vi "processSubDataPublish.vi"(8 "error in (no error)":errorcluster, 11 "MiddlewareSALThisComponent in":refnum<class "MiddlewareSALThisComponent.lvclass">) -> (0 "error out":errorcluster, 3 "MiddlewareSALThisComponent out":refnum<class "MiddlewareSALThisComponent.lvclass">)   [LabVIEW 2016, in "MiddlewareSALThisComponent.lvclass"]
uses:
  MiddlewareSALThisComponent.lvclass
  home/harini/tcs/ts_sedspectrometer/ComponentTemplateCore/ComponentModel/ComponentModel/Middleware/Middleware.lvclass
  ComponentTemplateCore/ComponentModel/ComponentModel/Middleware/Middleware.lvclass/Middleware.ctl
  ComponentTemplateCore/ComponentModel/ComponentModel/MiddlewareProcessEvent/MiddlewareProcessEvent.lvclass/MiddlewareProcessEvent.ctl
  MiddlewareSALThisComponent.lvclass/MiddlewareSALThisComponent.ctl
  PubSubDataEvent/PubSubDataEvent.lvclass/PubSubDataEvent.ctl
  <vilib>/Utility/error.llb/DialogType.ctl
  Typedefs/SubDataSignal.ctl
  ts_sallv_sedspectrometer/DataTypes/command_CaptureSpectImage.ctl
  ts_sallv_sedspectrometer/DataTypes/command_SetSpectTempSetpoint.ctl
  ts_sallv_sedspectrometer/DataTypes/command_StopImageCapture.ctl
  Typedefs/EXATypedefs.lvlib
  ComponentTemplateCore/ComponentModel/ComponentModel/Middleware/Middleware.lvclass
  ComponentTemplateCore/ComponentModel/ComponentModel/MiddlewareProcessEvent/MiddlewareProcessEvent.lvclass
  PubSubDataEvent/PubSubDataEvent.lvclass
  ProgrammaticInitialization/ProgrammaticInitialization.lvclass
  ts_sallv_sedspectrometer/SALLV_calibrationSpectrometer.lvlib
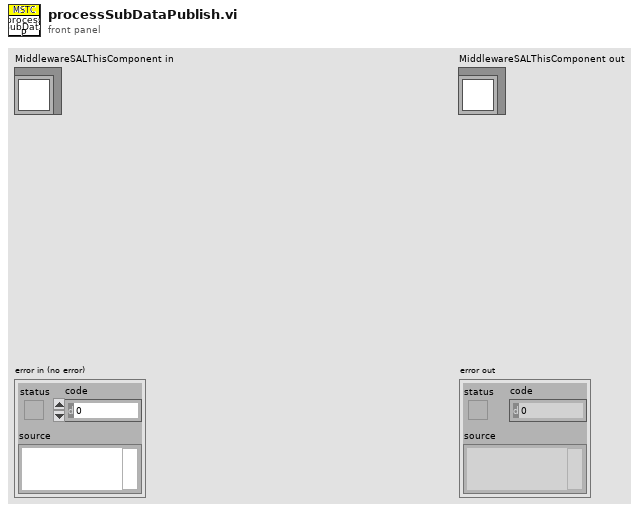
[diagram p1: front panel]
types:
  T1 = typedef "TypedefsDataEvents.lvlib/SubDataEvents.ctl" = cluster{"Disable":refnum<user-event>, "Enable":refnum<user-event>, "ExitControl":refnum<user-event>, "Standby":refnum<user-event>, "Heartbeat":refnum<user-event>, "Start":refnum<user-event>, "CaptureSpectImage":refnum<user-event>, "SetSpectTempSetpoint":refnum<user-event>, "StopImageCapture":refnum<user-event>}
  T2 = typedef "MiddlewareProcessEvents.ctl" = cluster{"disconnect":refnum<user-event>, "error":refnum<user-event>}
  T3 = typedef "EXATypedefs.lvlib/SubDataSignal.ctl" = enum16{"Disable", "Enable", "Exit", "GoToStandby", "HeartbeatIn", "Start", "CaptureSpectImage", "SetSpectTempSetpoint", "StopImageCapture"}
  T4 = typedef "SALLV_calibrationSpectrometer.lvlib/command_CaptureSpectImage.ctl" = cluster{"spectId":u16, "intTime":sgl, "intDelay":dbl, "numAverages":u16, "numScans":i32}
  T5 = typedef "SALLV_calibrationSpectrometer.lvlib/command_SetSpectTempSetpoint.ctl" = cluster{"spectId":u16, "setpoint":sgl}
  T6 = typedef "SALLV_calibrationSpectrometer.lvlib/command_StopImageCapture.ctl" = cluster{"SpectId":u16}
  T7 = typedef "DialogType.ctl" = u16
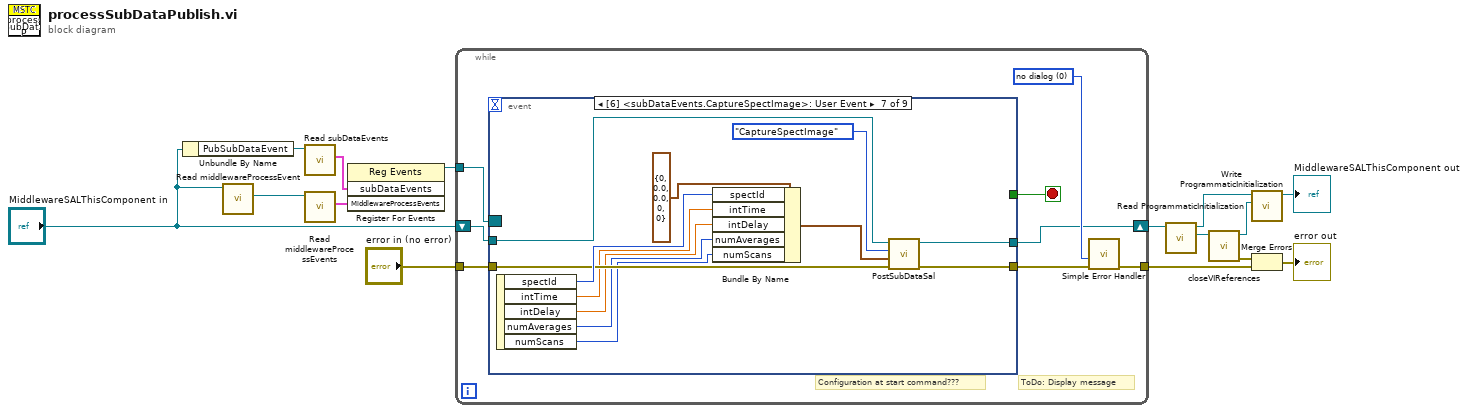
[diagram p0: block diagram]
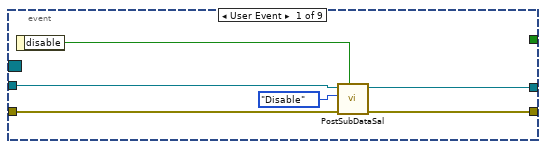
[diagram p2: hidden frame]
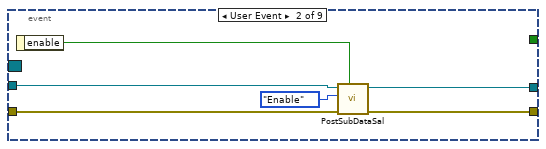
[diagram p3: hidden frame]
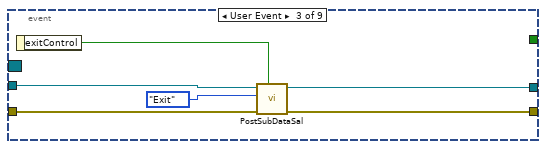
[diagram p4: hidden frame]
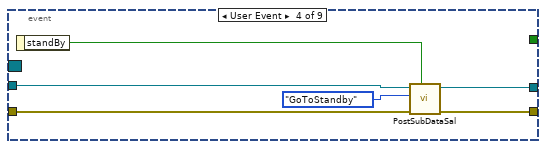
[diagram p5: hidden frame]
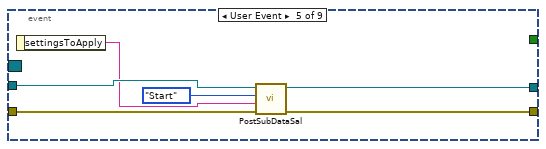
[diagram p6: hidden frame]
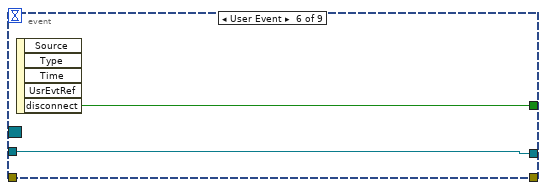
[diagram p7: hidden frame]
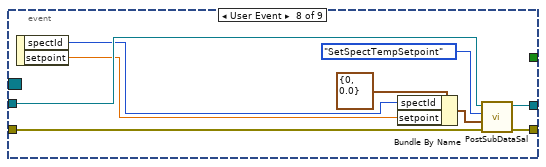
[diagram p8: hidden frame]
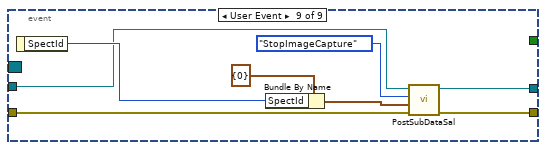
[diagram p9: hidden frame]
diagram:
  n1 = Unbundle By Name("MiddlewareSALThisComponent in") -> ("PubSubDataEvent"=w12:refnum<class "PubSubDataEvent.lvclass">)
  n2 = call "Read middlewareProcessEvent.vi"("Middleware in"="MiddlewareSALThisComponent in") -> ("middlewareProcessEvent"=w14:refnum<class "MiddlewareProcessEvent.lvclass">)  [unwired: 9 in, 1 out]
  n3 = call "Read subDataEvents.vi"("PubSubDataEvent in"=w12) -> ("subDataEvents"=w11:T1)  [unwired: 9 in, 1 out]
  n4 = call "Read middlewareProcessEvents.vi"("MiddlewareProcessEvent in"=w14) -> ("MiddlewareProcessEvents"=w13:T2)  [unwired: 9 in, 1 out]
  n5 = register-events(w11, w13) -> (reference out=w15:refnum<event-registration>)  [unwired: 2 in, 1 out]
  n6 = while {
    tunnel: w15 -> [w23]
    tunnel: "error in (no error)" -> [w20]
    tunnel: [w17] -> w1
    shift-right: [w16] -> w4
    shift-left: "MiddlewareSALThisComponent in" -> [w18]
    stop <- w22 stop-if-true
    w21 = T7 0 items=["no dialog", "OK message", "continue or stop message", "OK message + warnings", "continue/stop + warnings"] ("type of dialog (OK msg:1)")
    # "Configuration at start command???"
    # "ToDo: Display message"
    n7 = event shown="[6] <subDataEvents.CaptureSpectImage>: User Event" {
      selector: w23 -> [_ _ _ _ _ _ _ _ _]
      dyn-events: _ -> [_ _ _ _ _ _ _ _ _]
      timeout: _ -> [_ _ _ _ _ _ _ _ _]
      tunnel: [_ _ _ _ _ w55 _ _ _] -> w22
      tunnel: w20 -> [w28 w34 w38 w43 w52 _ w62 w70 w79]
      tunnel: [w29 w35 w41 w47 w53 _ w61 w69 w78] -> w19
      tunnel: w18 -> [w26 w32 w40 w46 w51 w54 w67 w76 w80]
      tunnel: [w24 w30 w36 w42 w48 w54 w60 w68 w77] -> w16
      event User Event {
        n8 = event-data() -> ("disable"=w25:bool)  [unwired: 1 in]
        n9 = call "PostSubDataSal.vi"("newValue (T)"=w25, "error in (no error)"=w28, "subDataSV"=SubDataSignal."Disable" ("SubDataSV"), "MiddlewareSALThisComponent in"=w26) -> ("error out"=w29:errorcluster, "MiddlewareSALThisComponent out"=w24:refnum<class "MiddlewareSALThisComponent.lvclass">)  [unwired: 6 in]
      }
      event User Event {
        n10 = event-data() -> ("enable"=w33:bool)  [unwired: 1 in]
        n11 = call "PostSubDataSal.vi"("newValue (T)"=w33, "error in (no error)"=w34, "subDataSV"=SubDataSignal."Enable" ("SubDataSV"), "MiddlewareSALThisComponent in"=w32) -> ("error out"=w35:errorcluster, "MiddlewareSALThisComponent out"=w30:refnum<class "MiddlewareSALThisComponent.lvclass">)  [unwired: 6 in]
      }
      event User Event {
        n12 = event-data() -> ("exitControl"=w37:bool)  [unwired: 1 in]
        n13 = call "PostSubDataSal.vi"("newValue (T)"=w37, "error in (no error)"=w38, "subDataSV"=SubDataSignal."Exit" ("SubDataSV"), "MiddlewareSALThisComponent in"=w40) -> ("error out"=w41:errorcluster, "MiddlewareSALThisComponent out"=w36:refnum<class "MiddlewareSALThisComponent.lvclass">)  [unwired: 6 in]
      }
      event User Event {
        n14 = event-data() -> ("standBy"=w45:bool)  [unwired: 1 in]
        n15 = call "PostSubDataSal.vi"("newValue (T)"=w45, "error in (no error)"=w43, "subDataSV"=SubDataSignal."GoToStandby" ("SubDataSV"), "MiddlewareSALThisComponent in"=w46) -> ("error out"=w47:errorcluster, "MiddlewareSALThisComponent out"=w42:refnum<class "MiddlewareSALThisComponent.lvclass">)  [unwired: 6 in]
      }
      event User Event {
        n16 = event-data() -> ("settingsToApply"=w49:string)  [unwired: 1 in]
        n17 = call "PostSubDataSal.vi"("error in (no error)"=w52, "value"=w49, "subDataSV"=SubDataSignal."Start" ("SubDataSV"), "MiddlewareSALThisComponent in"=w51) -> ("error out"=w53:errorcluster, "MiddlewareSALThisComponent out"=w48:refnum<class "MiddlewareSALThisComponent.lvclass">)  [unwired: 6 in]
      }
      event User Event {
        n18 = event-data() -> ("disconnect"=w55:bool)  [unwired: 1 in, 4 out]
      }
      event User Event {
        n19 = event-data() -> ("spectId"=w65:u16, "intTime"=w59:sgl, "intDelay"=w58:dbl, "numAverages"=w57:u16, "numScans"=w56:i32)  [unwired: 1 in]
        n20 = Bundle By Name(cluster=T4 {"spectId"=0, "intTime"=0.0, "intDelay"=0.0, "numAverages"=0, "numScans"=0} ("command_CaptureSpectImage"), "spectId"=w65, "intTime"=w59, "intDelay"=w58, "numAverages"=w57, "numScans"=w56) -> (w63:T4)
        n21 = call "PostSubDataSal.vi"("error in (no error)"=w62, "value"=w63, "subDataSV"=SubDataSignal."CaptureSpectImage", "MiddlewareSALThisComponent in"=w67) -> ("error out"=w61:errorcluster, "MiddlewareSALThisComponent out"=w60:refnum<class "MiddlewareSALThisComponent.lvclass">)  [unwired: 6 in]
      }
      event User Event {
        n22 = event-data() -> ("spectId"=w75:u16, "setpoint"=w74:sgl)  [unwired: 1 in]
        n23 = Bundle By Name(cluster=T5 {"spectId"=0, "setpoint"=0.0} ("command_SetSpectTempSetpoint"), "spectId"=w75, "setpoint"=w74) -> (w72:T5)
        n24 = call "PostSubDataSal.vi"("error in (no error)"=w70, "value"=w72, "subDataSV"=SubDataSignal."SetSpectTempSetpoint", "MiddlewareSALThisComponent in"=w76) -> ("error out"=w69:errorcluster, "MiddlewareSALThisComponent out"=w68:refnum<class "MiddlewareSALThisComponent.lvclass">)  [unwired: 6 in]
      }
      event User Event {
        n25 = event-data() -> ("SpectId"=w84:u16)  [unwired: 1 in]
        n26 = Bundle By Name(cluster=T6 {"SpectId"=0} ("command_StopImageCapture"), "SpectId"=w84) -> (w82:T6)
        n27 = call "PostSubDataSal.vi"("error in (no error)"=w79, "value"=w82, "subDataSV"=SubDataSignal."StopImageCapture", "MiddlewareSALThisComponent in"=w80) -> ("error out"=w78:errorcluster, "MiddlewareSALThisComponent out"=w77:refnum<class "MiddlewareSALThisComponent.lvclass">)  [unwired: 6 in]
      }
    }
    n28 = call <vilib>:"Simple Error Handler.vi"("type of dialog (OK msg:1)"=w21, "error in (no error)"=w19) -> ("error out"=w17:errorcluster)  [unwired: 3 in, 4 out]
  }
  n29 = call-dynamic "Read ProgrammaticInitialization.vi"("MiddlewareSALThisComponent in"=w4) -> ("ProgrammaticInitialization"=w8:refnum<class "ProgrammaticInitialization.lvclass">, "MiddlewareSALThisComponent out"=w7:refnum<class "MiddlewareSALThisComponent.lvclass">)  [unwired: 8 in, 1 out]
  n30 = call "closeVIReferences.vi"("ProgrammaticInitialization in"=w8) -> ("error out"=w3:errorcluster, "ProgrammaticInitialization out"=w6:refnum<class "ProgrammaticInitialization.lvclass">)  [unwired: 9 in]
  n31 = call-dynamic "Write ProgrammaticInitialization.vi"("ProgrammaticInitialization"=w6, "MiddlewareSALThisComponent in"=w7) -> ("MiddlewareSALThisComponent out"=→"MiddlewareSALThisComponent out":refnum<class "MiddlewareSALThisComponent.lvclass">)  [unwired: 8 in, 1 out]
  n32 = Merge Errors(w3, w1) -> (→"error out":errorcluster)
